vi "Variable Tree Build Shortcut Menu.vi"(8 "error in (no error)":errorcluster, 9 "Coords":T1, 10 "MenuRef":refnum<k9>, 11 "Variable Tree":refnum<vi>) -> (0 "error out":errorcluster)   [LabVIEW 2015, in "Project.lvclass"]
uses:
  Project.lvclass
  <vilib>/Utility/miscctls.llb/LVPoint32TypeDef.ctl
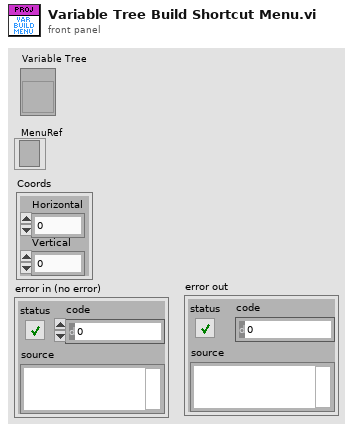
[diagram p1: front panel]
types:
  T1 = typedef "LVPoint32TypeDef.ctl" = cluster{"Horizontal":i32, "Vertical":i32}
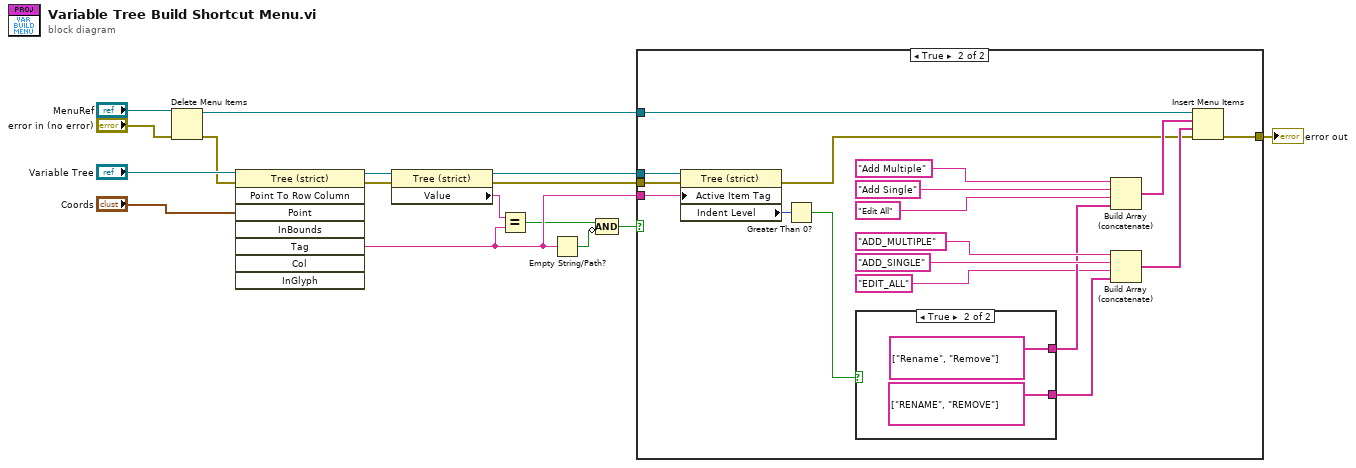
[diagram p0: block diagram]
diagram:
  n1 = Delete Menu Items(6:"error in (no error)", 9:"MenuRef") -> (0:w12:errorcluster, 3:w11:refnum<k9>)  [unwired: 2 in]
  n2 = invoke class="Tree (strict)" method="Point To Row Column"(reference="Variable Tree", error in=w12, "Point"="Coords") -> (reference out=w9:refnum<vi>, error out=w8:errorcluster, "Tag"=w6:string)  [unwired: 5 in, 5 out]
  n3 = property class="Tree (strict)"(reference=w9, error in=w8) -> (reference out=w1:refnum<vi>, error out=w2:errorcluster, "Value"=w7:string)
  n4 = Equal?(x=w7, y=w6) -> (x = y?=w5:bool)
  n5 = Empty String/Path?(string/path=w6) -> (empty?=w4:bool)
  n6 = Compound Arithmetic op=AND(w5, invert w4) -> (w3:bool)
  n7 = case shown="True" w3 {
    tunnel: w1 -> [_ w35]
    tunnel: w2 -> [w17 w34]
    tunnel: w6 -> [_ w27]
    tunnel: w11 -> [_ w32]
    tunnel: [w17 w31] -> w10
    frame False {
    }
    frame True {
      n8 = property class="Tree (strict)"(reference=w35, error in=w34, "Active Item Tag"=w27) -> (error out=w25:errorcluster, "Indent Level"=w33:i32)  [unwired: 1 out]
      n9 = Greater Than 0?(x=w33) -> (x > 0?=w26:bool)
      n10 = case shown="True" w26 {
        tunnel: [_ string[] ["Rename", "Remove"] ("item names")] -> w21
        tunnel: [_ string[] ["RENAME", "REMOVE"] ("item tags")] -> w19
        frame False {
        }
        frame True {
        }
      }
      n11 = Build Array (concatenate)("Add Multiple", "Add Single", "Edit All", w21) -> (w29:string[])
      n12 = Build Array (concatenate)("ADD_MULTIPLE", "ADD_SINGLE", "EDIT_ALL", w19) -> (w28:string[])
      n13 = Insert Menu Items(6:w25, 7:w28, 8:w29, 9:w32) -> (0:w31:errorcluster)  [unwired: 2 in, 2 out]
    }
  }
  "error out" <- w10
